vi "IPSHTBoxConfigRead.vi"(8 "error in (no error)":errorcluster, 11 "IP in":string) -> (0 "error out":errorcluster, 1 "status":bool, 2 "config":T1, 3 "IP out":string)   [LabVIEW 2018]
uses:
  <vilib>/httpClient/LabVIEWHTTPClient.lvlib
panel:
  out "body":string
  out "headers":string
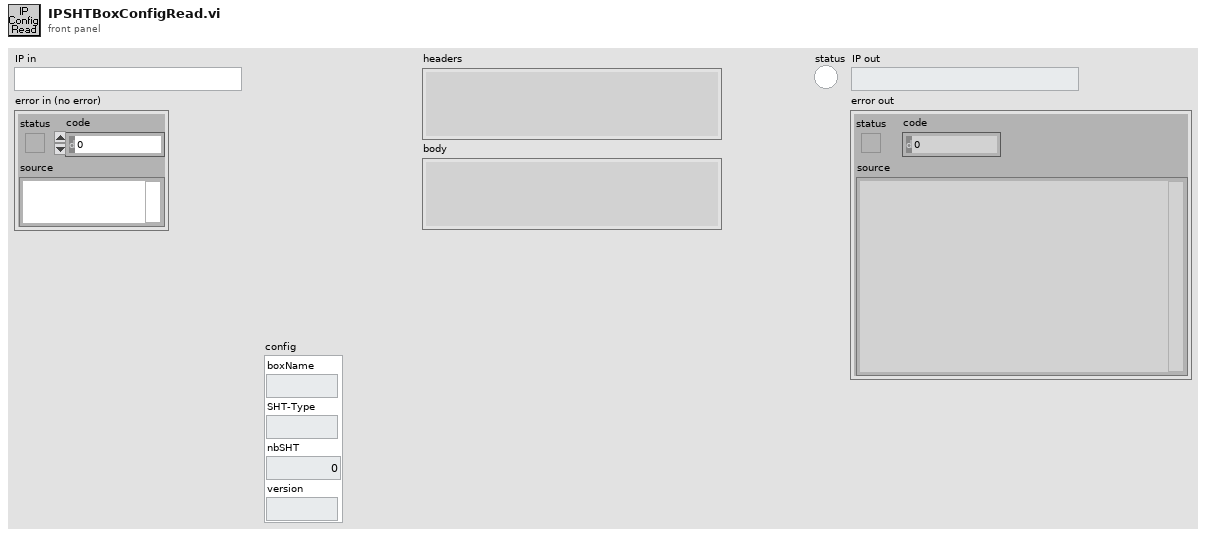
[diagram p1: front panel]
types:
  T1 = cluster{"boxName":string, "SHT-Type":string, "nbSHT":dbl, "version":string}
  T2 = cluster{"status":bool, "code":bool, "source":bool}
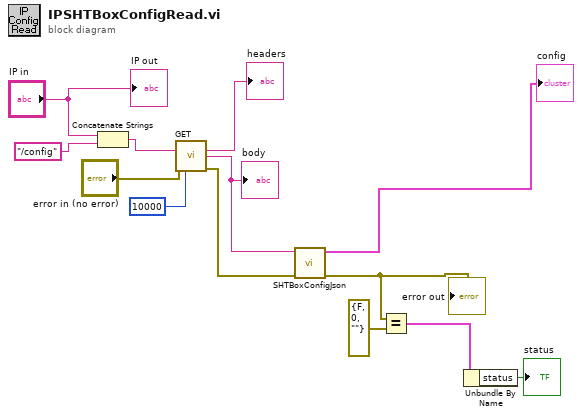
[diagram p0: block diagram]
diagram:
  n1 = Concatenate Strings("IP in", "/config" ("string")) -> (w9:string)
  n2 = call <vilib>:"GET.vi"("url"=w9, "error in (no error)"="error in (no error)", "timeout (10000)"=10000) -> ("headers"=→"headers":string, "body"=w12:string, "error out"=w7:errorcluster)  [unwired: 9 in, 1 out]
  "body" <- w12
  n3 = call "SHTBoxConfigJson.vi"("error in (no error)"=w7, "JSON string"=w12) -> ("error out"=w4:errorcluster, "value"=→"config":T1)  [unwired: 8 in]
  "error out" <- w4
  n4 = Equal?(x=w4, y=errorcluster {"status"=FALSE, "code"=0, "source"=""}) -> (x = y?=w2:T2)
  n5 = Unbundle By Name(w2) -> ("status"=→"status":bool)
  "IP out" <- "IP in"
